vi "LVCAM Nest Destroyed.vi"(9 "Nest Error":errorcluster, 10 "Nest Actor":refnum<class "LVCAM.lvclass">, 11 "Self Actor in":refnum<class "Self Actor.lvclass">) -> (0 "error out":errorcluster, 3 "Self Actor out":refnum<class "Self Actor.lvclass">)   [LabVIEW 2021, in "LVCAM.lvlib" / "Self Actor.lvclass"]
uses:
  Self Actor.lvclass
  LVCAM/LVCAM.lvclass
  Self Actor.lvclass/Self Actor.ctl
  Msgs/LVCAM Destroy Self/LVCAM Destroy Self Msg/LVCAM Destroy Self Msg.lvclass
  C:/PPLs/LabVIEW-Composed-Actor-Model-LVCAM/LabVIEW-Composed-Actor-Model-LVCAM/AAM/LVCAM/Msg/Msg.lvclass
  Self Msg Send.vi
  C:/PPLs/LabVIEW-Composed-Actor-Model-LVCAM/LabVIEW-Composed-Actor-Model-LVCAM/AAM/Msgs/LVCAM Destroy Self/LVCAM Destroy Self Msg/LVCAM Destroy Self Msg.lvclass
  C:/PPLs/LabVIEW-Composed-Actor-Model-LVCAM/LabVIEW-Composed-Actor-Model-LVCAM/AAM/Msgs/LVCAM Destroy Self/LVCAM Destroy Self/LVCAM Destroy Self.lvclass
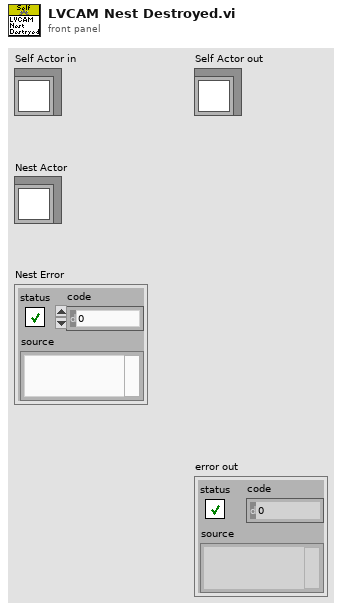
[diagram p1: front panel]
types:
  T1 = typedef "LVCAM.lvlib/Self Actor.lvclass/State.ctl" = enum16{"Safe Msging", "Destroying Self"}
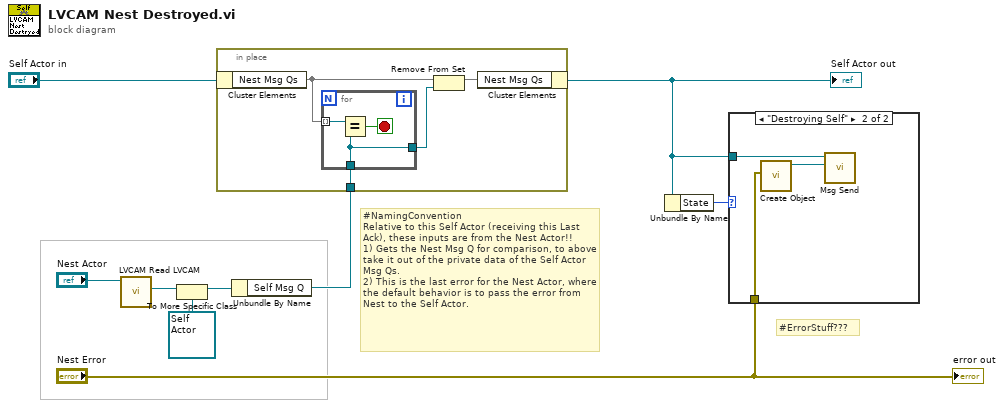
[diagram p0: block diagram]
diagram:
  # "#ErrorStuff???"
  # "#NamingConvention\nRelative to this Self Actor (receiving this Last Ack), these inputs are from the Nest Actor!! \n1) Gets the Nest Msg Q for comparison, to above take it out of the private data of the Self Actor Msg Qs.\n2) This is the last error for the Nest Actor, where the default behavior is to pass the error from Nest to the Self Actor."
  n1 = call-dynamic "LVCAM Read LVCAM.vi"("LVCAM Read LVCAM in"="Nest Actor") -> ("LVCAM"=w4:refnum<class "LVCAM.lvclass">)  [unwired: 10 in]
  n2 = To More Specific Class(target class=refnum<class "Self Actor.lvclass"> refnum ("Artifex Actor Model.lvlib:Self Actor.lvclass"), reference=w4) -> (specific class reference=w9:refnum<class "Self Actor.lvclass">)  [unwired: 1 in, 1 out]
  n3 = Unbundle By Name(w9) -> ("Self Msg Q"=w6:refnum<class "Msg Q.lvclass">)
  n4 = in-place {
    in-place-border: w6 -> [w11]
    n5 = in-place-cluster #1("Self Actor in") -> ("Nest Msg Qs"=w13:set{refnum<class "Msg Q.lvclass">})
    n6 = for {
      tunnel: w11 -> [w14]
      tunnel: w13 -> [w15] mode=indexing
      tunnel: [w14] -> w10
      stop <- w16 stop-if-true
      n7 = Equal?(x=w15, y=w14) -> (x = y?=w16:bool)
    }
    n8 = Remove From Set(10:w10, 11:w13) -> (3:w12:set{refnum<class "Msg Q.lvclass">})  [unwired: 1 out]
    n9 = in-place-cluster #1("Nest Msg Qs"=w12) -> (w2:refnum<class "Self Actor.lvclass">)
  }
  "Self Actor out" <- w2
  n10 = Unbundle By Name(w2) -> ("State"=w3:T1)
  n11 = case shown="\"Destroying Self\"" w3 {
    tunnel: w2 -> [_ w18]
    tunnel: "Nest Error" -> [_ w17]
    frame "Safe Msging" {
    }
    frame "Destroying Self" {
      n12 = call "Create Object.vi"("Error"=w17) -> ("LVCAM Destroy Self Msg out"=w19:refnum<class "LVCAM Destroy Self Msg.lvclass">)  [unwired: 10 in]
      n13 = call-poly "Msg Send.vi"("Msg"=w19, "Self Actor in"=w18) -> ()  [unwired: 9 in, 1 out]
    }
  }
  "error out" <- "Nest Error"
